vi "실습 4-3 배열 인덱스 함수.vi"() -> ()   [LabVIEW 2014]
panel:
  out "원소 2":i32
  out "부분배열 4":i32[](array[numeric])
  out "부분배열 3":i32[](array[numeric])
  out "부분배열 2":i32[](array[numeric])
  out "부분배열":i32[](array[numeric])
  out "원소":i32
  out "배열":i32[][](array[numeric])
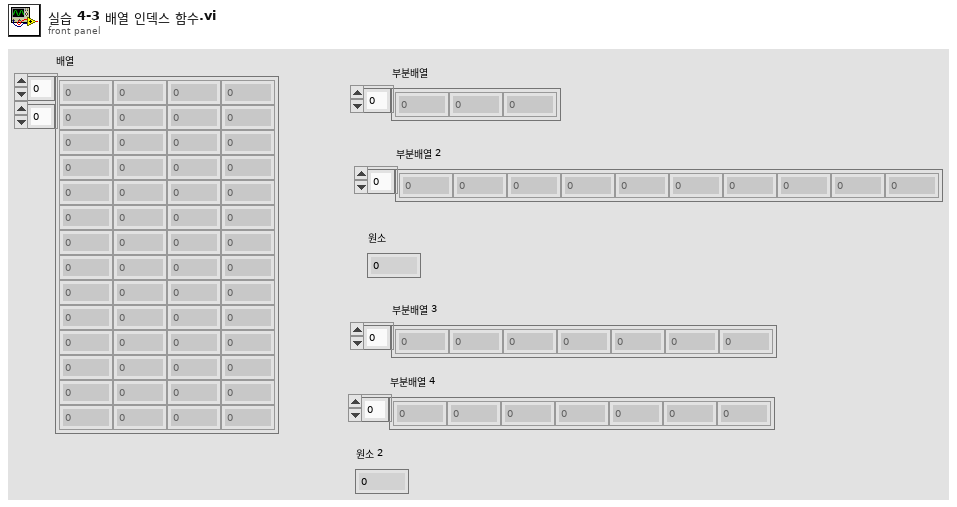
[diagram p1: front panel]
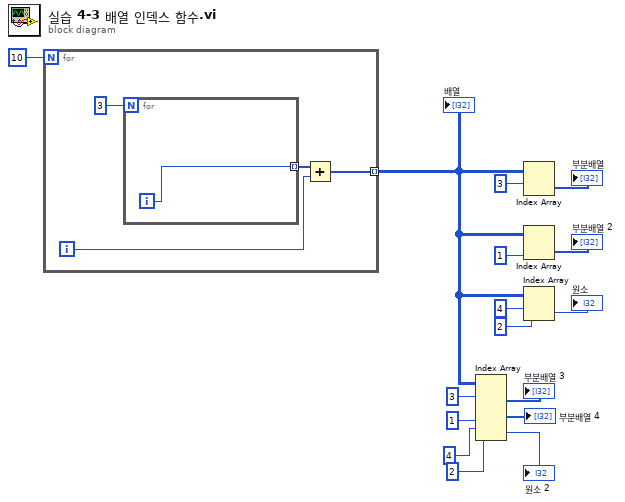
[diagram p0: block diagram]
diagram:
  n1 = for {
    N: 10 -> [_]
    tunnel: [w17] -> w8 mode=indexing
    i -> [w18]
    n2 = for {
      N: 3 -> [_]
      tunnel: [w21] -> w19 mode=indexing
      i -> [w21]
    }
    n3 = Add(x=w19, y=w18) -> (x+y=w17:i32[])
  }
  "배열" <- w8
  n4 = Index Array(array=w8, index (row) #1=3 ("인덱스 (행)"), index (col) #2=1 ("비활성화된 인덱스 (열)"), index (row) #3=4 ("인덱스 (행)"), index (col) #3=2 ("비활성화된 인덱스 (행)")) -> (element #1=→"부분배열 3":i32[], element #2=→"부분배열 4":i32[], element #3=→"원소 2":i32)  [unwired: 2 in]
  n5 = Index Array(array=w8, index (row)=3 ("인덱스 (행)")) -> (element=→"부분배열":i32[])  [unwired: 1 in]
  n6 = Index Array(array=w8, index (col)=1 ("비활성화된 인덱스 (열)")) -> (element=→"부분배열 2":i32[])  [unwired: 1 in]
  n7 = Index Array(array=w8, index (row)=4 ("인덱스 (행)"), index (col)=2 ("비활성화된 인덱스 (열)")) -> (element=→"원소":i32)
